vi "OpenScan-20170126-FPGA.vi"() -> ()   [LabVIEW 2015]
uses:
  <vilib>/Platform/TimedLoop/XDataNode/XDataNode.xnode
  <vilib>/Platform/TimedLoop/XDataNode/nitl_modes.ctl
  <vilib>/Platform/TimedLoop/XDataNode/XDNodeRunTimeDep.lvlib
  <vilib>/Platform/TimedLoop/XDataNode/wakeup.ctl
  <vilib>/Platform/TimedLoop/XDataNode/timing_clust.ctl
  <vilib>/rvi/DataTransferAndStorage/Container/XNode/niFpgaContainer.xnode
  <vilib>/eio/EIONode/EIONode.xnode
  <vilib>/rvi/eio/common/nirviEmuTemplateMethod_errors.vi
  <vilib>/rvi/interface/RandomDataEmulation/nirviRandomDataFpgaReadWriteTemplate.vi
  <vilib>/rvi/Memory/Memory_Emulation/niFpgaMemoryEmulationDramWriteAndRequestData.vi
  <vilib>/rvi/Memory/Memory_Emulation/niFpgaMemoryFastEmulationDramWriteAndRequestData.vi
  <vilib>/rvi/Memory/Memory_Emulation/niFpgaMemoryEmulationDramRetrieveData.vi
  <vilib>/rvi/LocalResourceManager/LocalResourceManager.xnode
  <vilib>/rvi/DataTransferAndStorage/Container/Common/niFpgaContainerGetUniqueNameForEmu.vi
  <vilib>/rvi/DataTransferAndStorage/Container/Common/niFpgaContainerSetEmuInfo.vi
  <vilib>/rvi/eio/common/nirviEmuReportErrorAndStop.vi
  <vilib>/rvi/FIFO/Fifo_Resource/nirvififoEmulationRead.vi
  <vilib>/rvi/FIFO/Fifo_Resource/nirvififoEmulationWrite.vi
  <vilib>/rvi/FIFO/Fifo_Resource/nirvififoEmulationClear.vi
panel:
  out "Scan rate(ticks)":u32
  out "loop count":i32
  out "Averaged data address":u32
  out "Averaged image displayed?":bool
  out "Image averaging done?":bool
  in  "Kalman gain":fxp<+,16,1>=0.1015625
  in  "Filter gain":fxp<+,16,0>=0.8000030517578125
  out "Pixel clock":bool
  out "Line clock":bool
  out "Next frame?":bool
  out "Display_frames done":i32
  out "Waveform output frames done":i32
  out "Acquisition frames done":i32
  in  "Frame retrace time":u32 caption="Frame retrace time (ms)"
  out "All waveform output finish?":bool
  in  "Imaging mode":i16(ring)=2 items=["Grab, single frame", "Focus, infinite frames", "Loop, finite frames"]
  in  "Num of frames":i32
  out "Frame Galvo signal write done?":bool
  in  "Total elements":u32
  out "Frame address":u32
  in  "Write Frame Galvo signal?":bool
  in  "max addr":u32=1024
  out "Write DRAM done?":bool
  in  "Write DRAM enable?":bool
  out "Imaging data address":u32
  out "Frame imaging data displayed?":bool
  out "Frame acquisition finish?":bool
  in  "Samples per frame":u32
  in  "Pixel pulse_initial delay":i32
  out "Samples acquired":u32
  in  "Pixel clock_pulse width(tick)":i32
  in  "Resolution":i32
  in  "Num of undershoot":i32
  in  "Elements per line":i32
  out "Request address":u32
  out "Galvo signal readed":u32
  out "Frame waveform output finish?":bool
  out "Data":u32
  in  "Num of elements":u32
  in  "Pixel time (tick)":i32
  # "Waveform generation"
  # "Acquisition"
  # "Kalman filter and image diaplay"
  # "This vi is the FPGA vi for a laser scanning microscope working under photon conuting mode. It \ncontrols scan waveform generation, sychronized data acquisition, Kalman filter of imaging data,\nand transfer processed data to PC for display."
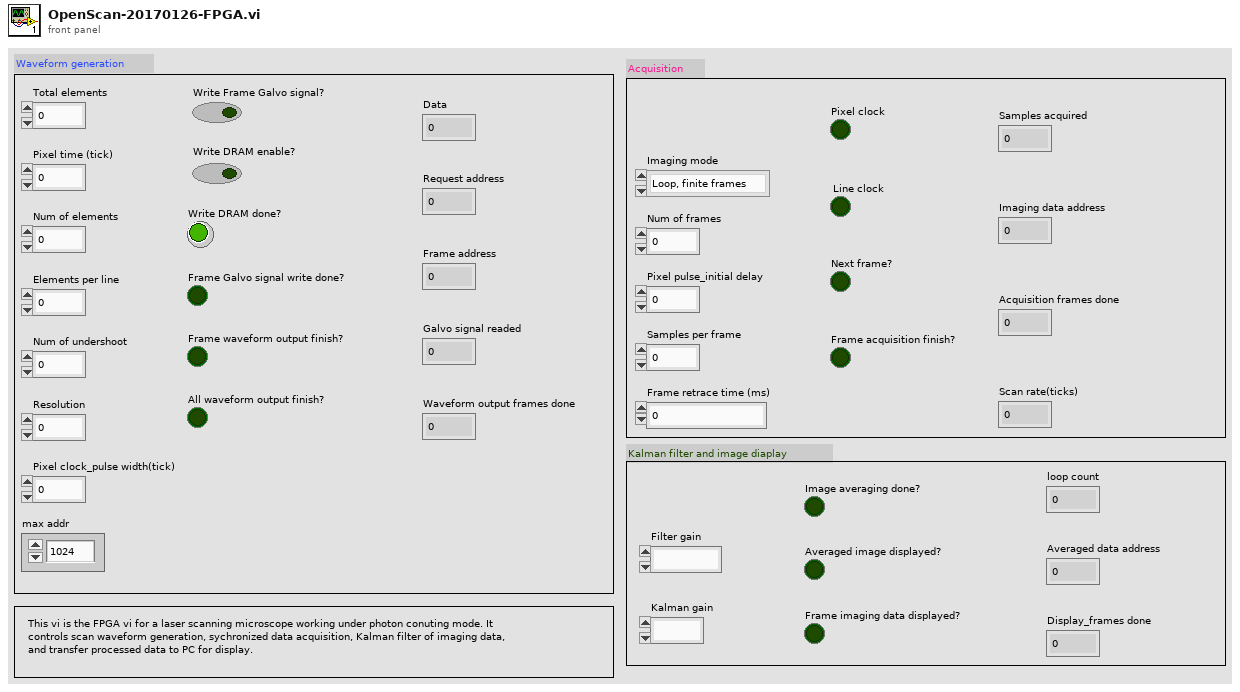
[diagram p1: front panel]
types:
  T1 = typedef "XDNodeRunTimeDep.lvlib/timing_clust.ctl" = cluster{"Expected End [f-1]":u64, "Actual End [f-1]":u64, "Finished Late? [f-1]":bool, "Expected End [i-1]":u64, "Actual End [i-1]":u64, "Finished Late? [i-1]":bool, "Expected Start [i]":u64, "Actual Start [i]":u64, "Expected Start [f]":u64, "Actual Start [f]":u64, "Source Name":string, "Structure Name":string, "Period":i64, "Deadline":i64, "Offset":i64, "Start":i64, "Priority":i32, "Timeout":i32, "Mode":T2, "Wakeup Reason":T3, "Error":errorcluster, "Source Type":string, "Secondary Source Type":string, "Global End Time":u64, "Global Start Time":u64, "Frame Duration":u64, "Iteration Duration":u64, "Assigned CPU":i32, "I/O Scan Engine Mode":u32}
  T2 = typedef "XDNodeRunTimeDep.lvlib/nitl_modes.ctl" = enum32{"No Change", "Process missed periods, maintain original phase", "Discard missed periods, maintain original phase", "Process missed periods, ignore original phase", "Discard missed periods, ignore original phase"}
  T3 = typedef "XDNodeRunTimeDep.lvlib/wakeup.ctl" = enum32{"Normal", "Aborted", "Asynchronous wakeup", "Timing source error", "Timed loop error", "Timeout"}
  T4 = cluster{"Numeric 1":u32, "Numeric 2":u32, "Numeric 3":u32, "Numeric 4":u32, "Numeric 5":u32, "Numeric 6":u32, "Numeric 7":u32, "Numeric 8":u32, "Numeric 9":u32, "Numeric 10":u32, "Numeric 11":u32, "Numeric 12":u32, "Numeric 13":u32, "Numeric 14":u32, "Numeric 15":u32, "Numeric 16":u32}
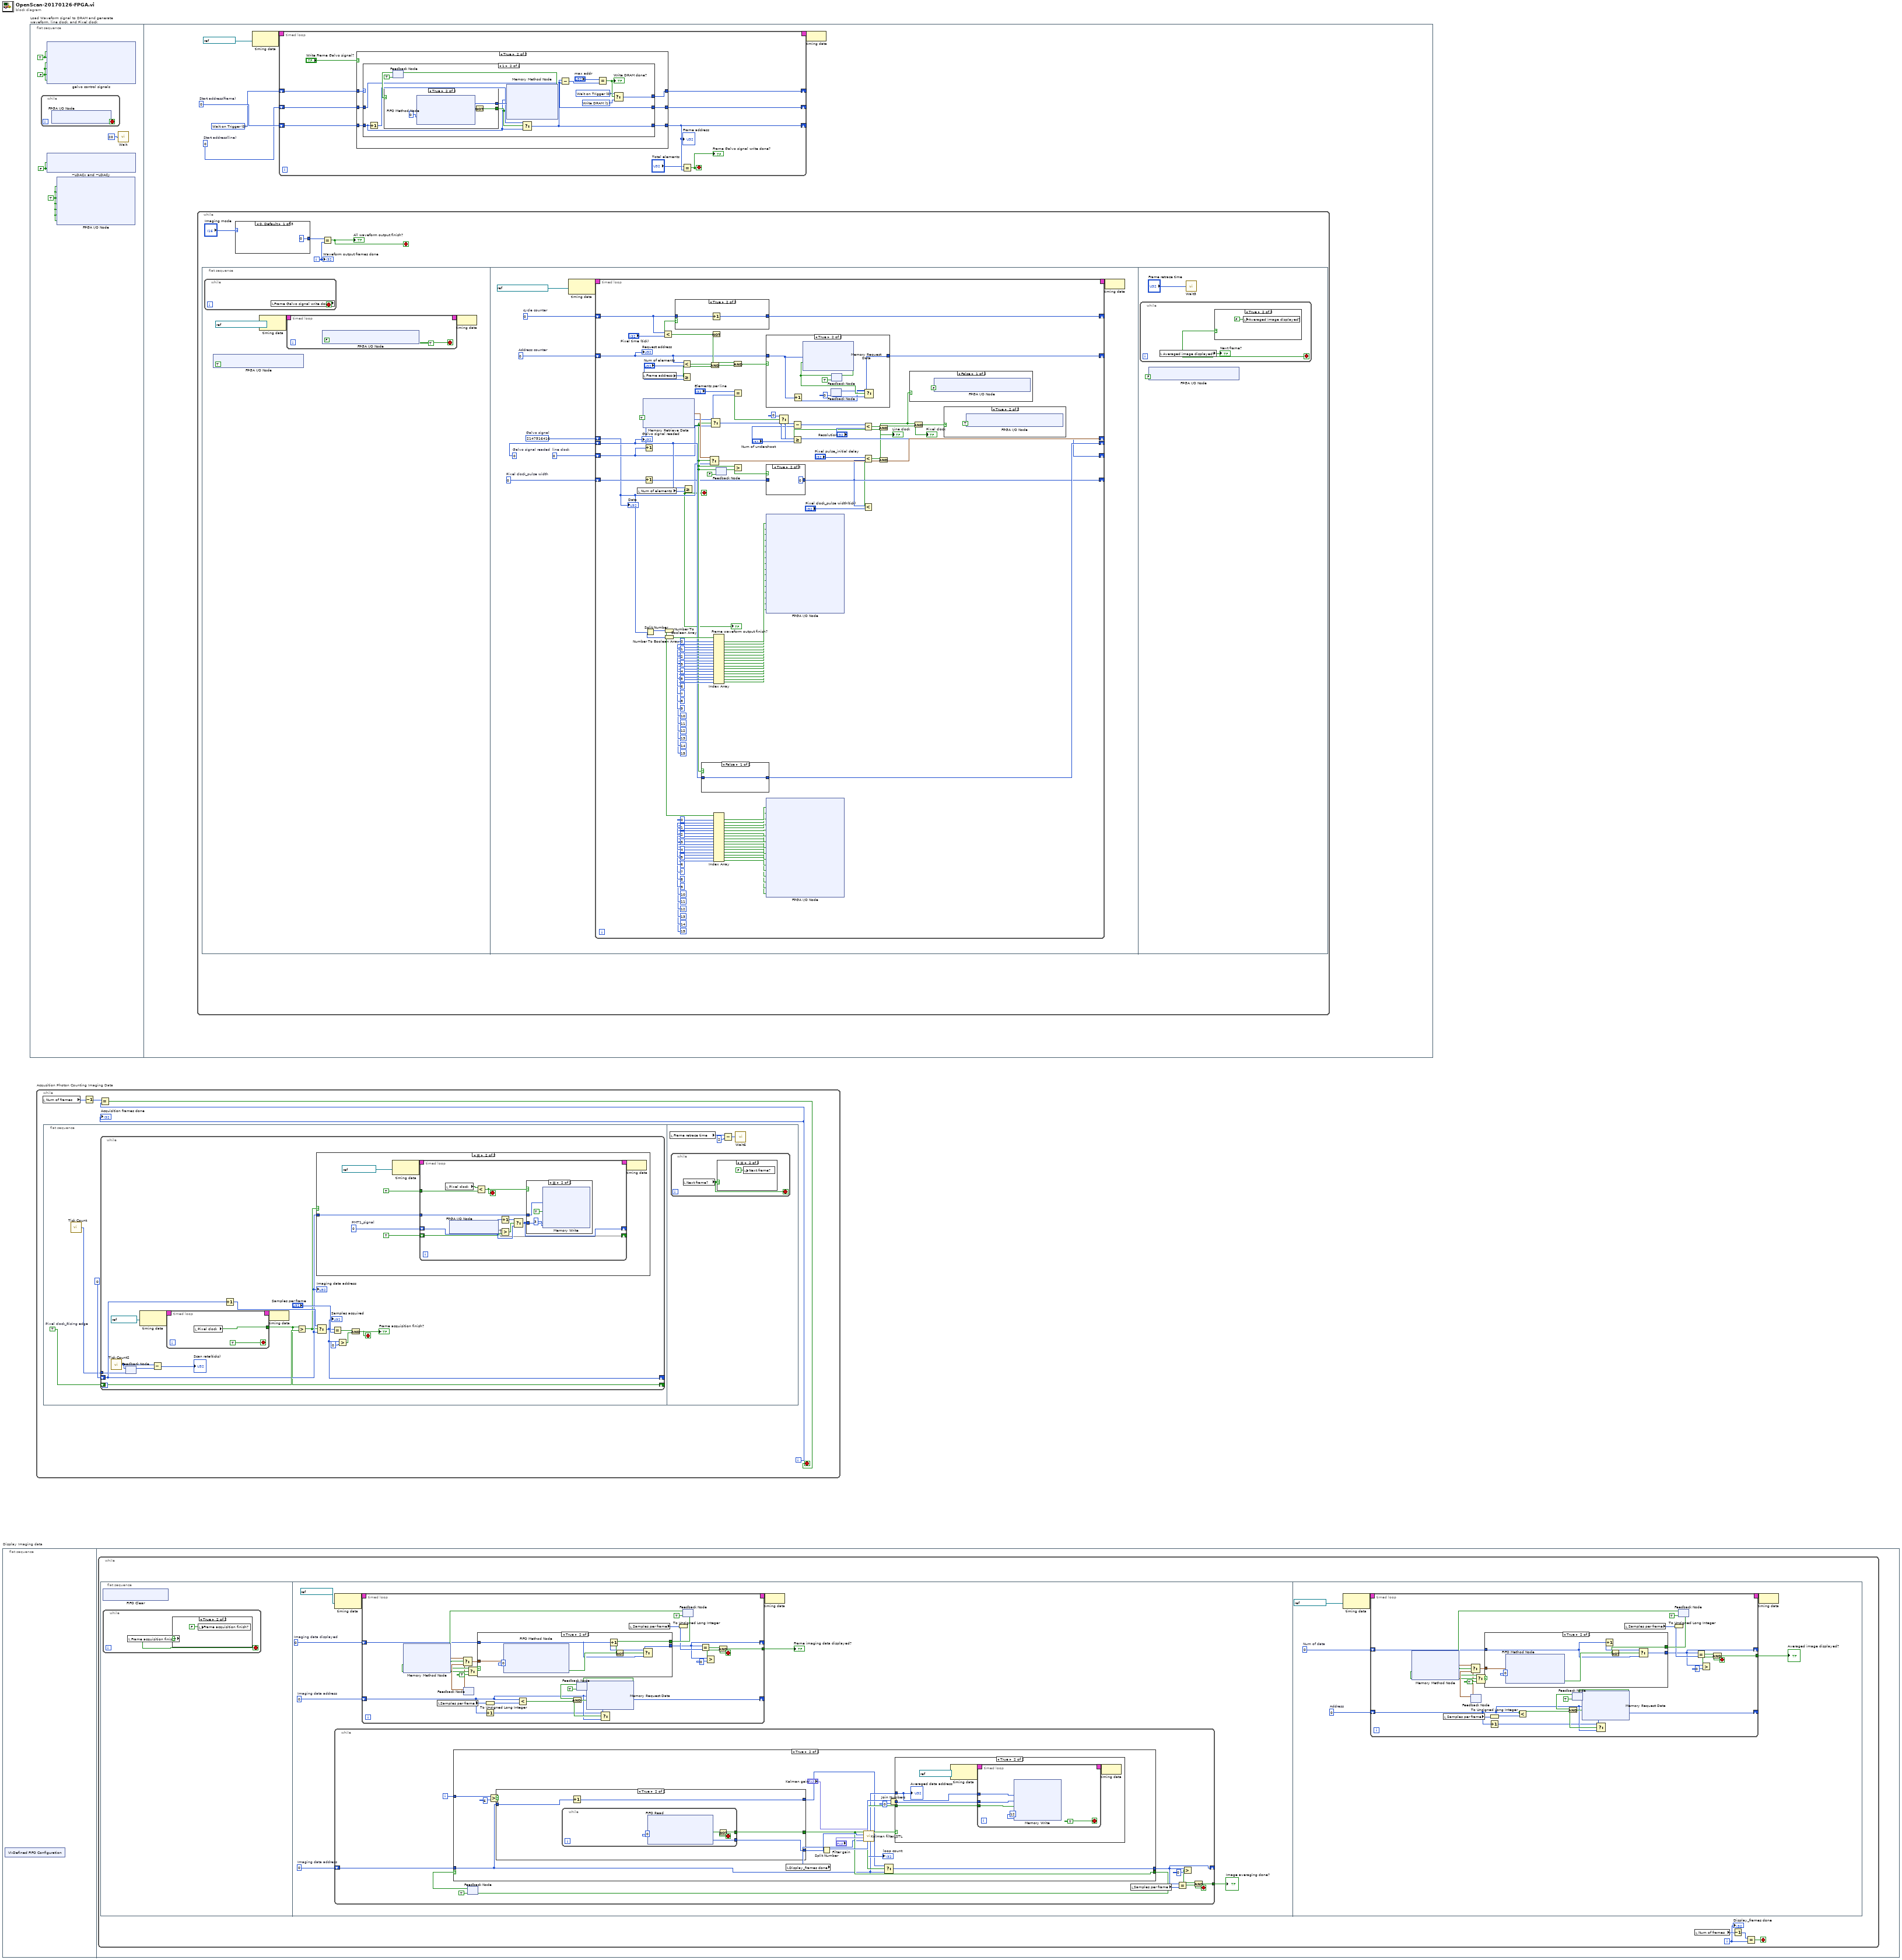
[diagram p0: block diagram]
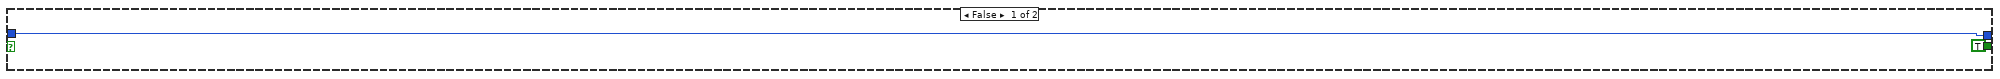
[diagram p6: hidden frame]
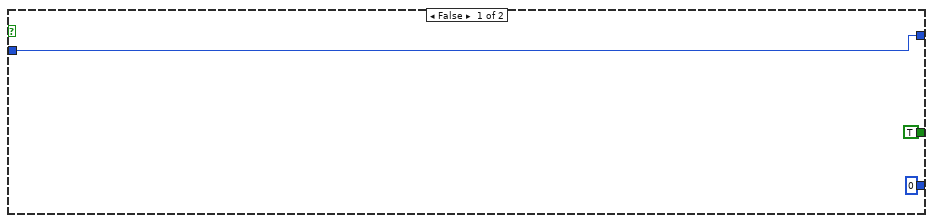
[diagram p7: hidden frame]
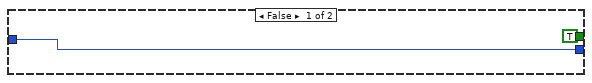
[diagram p9: hidden frame]
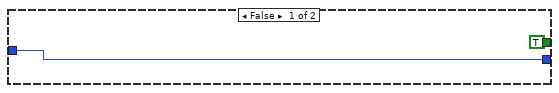
[diagram p10: hidden frame]
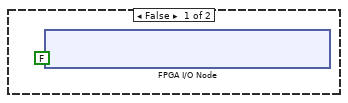
[diagram p11: hidden frame]
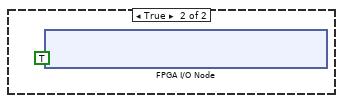
[diagram p13: hidden frame]
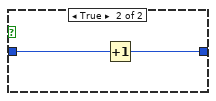
[diagram p14: hidden frame]
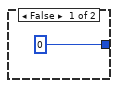
[diagram p16: hidden frame]
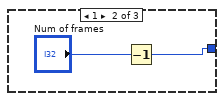
[diagram p18: hidden frame]
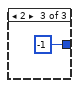
[diagram p19: hidden frame]
diagram:
  n1 = flat-sequence "Display Imaging data" {
    frame #0 {
      n2 = xnode "VI-Defined FIFO Configuration"() -> ()  [unwired: 1 out]
    }
    frame #1 {
      n3 = while {
        i -> [w1]
        stop <- w3 stop-if-true
        n4 = flat-sequence {
          frame #0 {
            n5 = xnode ("FIFO Clear")() -> ()  [unwired: 1 in, 1 out]
            n6 = while {
              stop <- w5 stop-if-true
              n7 = local read "Frame acquisition finish?"() -> (w5:bool)
              n8 = case shown="True" w5 {
                frame False {
                }
                frame True {
                  n9 = local write "Frame acquisition finish?"(FALSE ("Frame acquisition finish?")) -> ()
                }
              }
            }
          }
          frame #1 {
            w8 = u32 0  # Imaging data address
            w11 = u32 0  # Imaging data displayed
            w12 = u32 0  # Imaging data address
            n10 = node-c288(refnum<k21> "DRAM Clock" ("Source Name")) -> (w14:T1)
            n11 = while {
              shift-right: [w21] -> _
              shift-left: w8 -> [w23]
              tunnel: [w18] -> w7
              i -> [w15]
              stop <- w18 stop-if-true
              n12 = feedback #1(TRUE ("Timed Out?")) -> (w24:bool)
              n13 = case shown="True" w24 {
                tunnel: [TRUE ("Timed Out?") w35] -> w25
                tunnel: w23 -> [w26 w29]
                tunnel: [w26 w41] -> w21
                tunnel: w15 -> [_ w32]
                frame False {
                }
                frame True {
                  n14 = Greater?(x=w32, y=6) -> (0:w30:bool)
                  n15 = case shown="True" w30 {
                    tunnel: [u32 0 ("Element") w52] -> w45
                    tunnel: [TRUE w51] -> w35
                    tunnel: w29 -> [w48 w50]
                    tunnel: [w48 w49] -> w28
                    frame False {
                    }
                    frame True {
                      n16 = while {
                        tunnel: [w53] -> w51
                        tunnel: [w54] -> w52
                        stop <- w53 stop-if-true
                        n17 = xnode ("FIFO Read")("超时"=0 ("Timeout")) -> ("元素"=w54:u32, "超时？"=w55:bool)  [unwired: 1 in, 1 out]
                        n18 = Not(x=w55) -> (.not. x?=w53:bool)
                      }
                      n19 = Increment(x=w50) -> (x+1=w49:u32)
                    }
                  }
                  n20 = local read "Display_frames done"() -> (w33:i32)
                  n21 = Split Number(x=w45) -> (hi(x)=w40:u16, lo(x)=w43:u16)
                  n22 = call "Kalman filter_STL.vi"("Previous predicted pixel value"=w40, "Kalman gain"="Kalman gain", "Frame number"=w33, "Filter gain"="Filter gain", "Pixel value"=w43, "Input valid"=w35) -> ("Kalman filter result"=w38:u16, "loop count"=→"loop count":i32, "output valid"=w36:bool)  [unwired: 3 in]
                  n23 = Select(t=w28, s=w36, f=w29) -> (s? t:f=w41:u32)
                  n24 = Join Numbers(hi=w38, lo=u16 0) -> ((hi.lo)=w39:u32)
                  n25 = case shown="True" w36 {
                    tunnel: w36 -> [_ w60]
                    tunnel: w29 -> [_ w59]
                    tunnel: w39 -> [_ w57]
                    frame False {
                    }
                    frame True {
                      n26 = node-c288(refnum<k21> "DRAM Clock" ("Source Name")) -> (w62:T1)
                      n27 = timed-loop {
                        timing: w62 -> [_]
                        timing-out: [_] -> w61
                        tunnel: w57 -> [w67]
                        tunnel: w60 -> [w66]
                        tunnel: w59 -> [w65]
                        stop <- TRUE stop-if-true
                        n28 = xnode ("Memory Write")("地址"=w65, "数据"=w67, "输入有效"=w66, "字节启用"=i64 12 ("Byte Enables")) -> ()  [unwired: 1 in, 2 out]
                      }
                      n29 = node-c288(w61) -> ()
                      "Averaged data address" <- w59
                    }
                  }
                }
              }
              n30 = feedback-in #1(w25) -> ()
              n31 = local read "Samples per frame"() -> (w17:u32)
              n32 = Equal?(x=w21, y=w17) -> (x = y?=w19:bool)
              n33 = Greater?(x=w21, y=u32 0) -> (0:w20:bool)
              n34 = And(x=w20, y=w19) -> (x .and. y?=w18:bool)
            }
            "Image averaging done?" <- w7
            n35 = timed-loop {
              shift-right: [w93] -> _
              shift-left: w12 -> [w95]
              timing: w14 -> [_]
              timing-out: [_] -> w13
              shift-right: [w80] -> _
              shift-left: w11 -> [w83]
              tunnel: [w75] -> w9
              stop <- w75 stop-if-true
              n36 = local read "Samples per frame"() -> (w100:u32)
              n37 = feedback #2() -> (w87:T4)  [unwired: 1 in]
              n38 = To Unsigned Long Integer(number=w100) -> (unsigned 32bit integer=w82:u32)
              n39 = Increment(x=w95) -> (x+1=w94:u32)
              n40 = Less?(x=w95, y=w82) -> (x < y?=w99:bool)
              n41 = feedback #3(TRUE ("Ready for Input")) -> (w97:bool)
              n42 = And(x=w97, y=w99) -> (x .and. y?=w96:bool)
              n43 = xnode ("Memory Request Data")("地址"=w95, "输入有效"=w96) -> ("输入就绪"=w98:bool)  [unwired: 1 in, 1 out]
              n44 = feedback-in #3(w98) -> ()
              n45 = Select(t=w94, s=w96, f=w95) -> (s? t:f=w93:u32)
              n46 = local read "Samples per frame"() -> (w92:u32)
              n47 = To Unsigned Long Integer(number=w92) -> (unsigned 32bit integer=w81:u32)
              n48 = feedback #4(TRUE) -> (w86:bool)
              n49 = xnode ("Memory Method Node")("输出就绪"=w86) -> ("数据"=w91:T4, "输出有效"=w84:bool)  [unwired: 1 in, 1 out]
              n50 = Select(t=w91, s=w86, f=w87) -> (s? t:f=w74:T4)
              n51 = feedback-in #2(w74) -> ()
              n52 = Select(t=w84, s=w86, f=TRUE) -> (s? t:f=w90:bool)
              n53 = case shown="True" w90 {
                tunnel: [TRUE w106] -> w89
                tunnel: w74 -> [_ w103]
                tunnel: w83 -> [w101 w105]
                tunnel: [w101 w104] -> w80
                frame False {
                }
                frame True {
                  n54 = xnode ("FIFO Method Node")("元素"=w103, "超时"=0 ("Timeout")) -> ("超时？"=w108:bool)  [unwired: 1 in, 1 out]
                  n55 = Increment(x=w105) -> (x+1=w107:u32)
                  n56 = Not(x=w108) -> (.not. x?=w106:bool)
                  n57 = Select(t=w107, s=w106, f=w105) -> (s? t:f=w104:u32)
                }
              }
              n58 = feedback-in #4(w89) -> ()
              n59 = Equal?(x=w80, y=w81) -> (x = y?=w77:bool)
              n60 = Greater?(x=w80, y=u32 0) -> (0:w78:bool)
              n61 = And(x=w77, y=w78) -> (x .and. y?=w75:bool)
            }
            "Frame imaging data displayed?" <- w9
            n62 = node-c288(w13) -> ()
          }
          frame #2 {
            w118 = u32 0  # Address
            w119 = u32 0  # Num of data
            n63 = node-c288(refnum<k21> "DRAM Clock" ("Source Name")) -> (w121:T1)
            n64 = timed-loop {
              shift-right: [w141] -> _
              shift-left: w118 -> [w143]
              timing: w121 -> [_]
              timing-out: [_] -> w120
              shift-right: [w128] -> _
              shift-left: w119 -> [w131]
              tunnel: [w123] -> w117
              stop <- w123 stop-if-true
              n65 = local read "Samples per frame"() -> (w148:u32)
              n66 = feedback #5() -> (w135:T4)  [unwired: 1 in]
              n67 = To Unsigned Long Integer(number=w148) -> (unsigned 32bit integer=w130:u32)
              n68 = Increment(x=w143) -> (x+1=w142:u32)
              n69 = Less?(x=w143, y=w130) -> (x < y?=w147:bool)
              n70 = feedback #6(TRUE ("Ready for Input")) -> (w145:bool)
              n71 = And(x=w145, y=w147) -> (x .and. y?=w144:bool)
              n72 = xnode ("Memory Request Data")("地址"=w143, "输入有效"=w144) -> ("输入就绪"=w146:bool)  [unwired: 1 in, 1 out]
              n73 = feedback-in #6(w146) -> ()
              n74 = Select(t=w142, s=w144, f=w143) -> (s? t:f=w141:u32)
              n75 = local read "Samples per frame"() -> (w140:u32)
              n76 = To Unsigned Long Integer(number=w140) -> (unsigned 32bit integer=w129:u32)
              n77 = feedback #7(TRUE) -> (w134:bool)
              n78 = xnode ("Memory Method Node")("输出就绪"=w134) -> ("数据"=w139:T4, "输出有效"=w132:bool)  [unwired: 1 in, 1 out]
              n79 = Select(t=w139, s=w134, f=w135) -> (s? t:f=w122:T4)
              n80 = feedback-in #5(w122) -> ()
              n81 = Select(t=w132, s=w134, f=TRUE) -> (s? t:f=w138:bool)
              n82 = case shown="True" w138 {
                tunnel: [TRUE w154] -> w137
                tunnel: w122 -> [_ w151]
                tunnel: w131 -> [w149 w153]
                tunnel: [w149 w152] -> w128
                frame False {
                }
                frame True {
                  n83 = xnode ("FIFO Method Node")("元素"=w151, "超时"=0 ("Timeout")) -> ("超时？"=w156:bool)  [unwired: 1 in, 1 out]
                  n84 = Increment(x=w153) -> (x+1=w155:u32)
                  n85 = Not(x=w156) -> (.not. x?=w154:bool)
                  n86 = Select(t=w155, s=w154, f=w153) -> (s? t:f=w152:u32)
                }
              }
              n87 = feedback-in #7(w137) -> ()
              n88 = Equal?(x=w128, y=w129) -> (x = y?=w125:bool)
              n89 = Greater?(x=w128, y=u32 0) -> (0:w126:bool)
              n90 = And(x=w125, y=w126) -> (x .and. y?=w123:bool)
            }
            "Averaged image displayed?" <- w117
            n91 = node-c288(w120) -> ()
          }
        }
        n92 = local read "Num of frames"() -> (w4:i32)
        n93 = Decrement(x=w4) -> (x-1=w2:i32)
        n94 = Equal?(x=w2, y=w1) -> (x = y?=w3:bool)
        "Display_frames done" <- w1
      }
    }
  }
  n95 = flat-sequence "Load Waveform signal to DRAM and generate waveform, line clock, and Pixel clock" {
    frame #0 {
      w166 = FALSE ("_LDACx")
      w168 = FALSE ("_CSx")
      w167 = TRUE ("_CLRx")
      w164 = TRUE ("IO Module\\DDCA_DIO8-15_WE")
      n96 = while {
        stop <- w169 stop-if-true
        n97 = xnode "FPGA I/O Node"() -> ("IO Module IO Enabled"=w169)  [unwired: 1 in, 1 out]
      }
      n98 = xnode "galvo control signals"("IO Module\\CLRx(DDCB_DIO0_WRITE)"=w167, "IO Module\\CLRy(DDCB_DIO1_WRITE)"=w167, "IO Module\\CSx(DDCB_DIO2_WRITE)"=w168, "IO Module\\CSy(DDCB_DIO3_WRITE)"=w168, "IO Module\\R_Wx(DDCB_DIO4_WRITE)"=w168, "IO Module\\R_Wy(DDCB_DIO5_WRITE)"=w168) -> ()  [unwired: 6 in, 6 out]
      n99 = xnode "~LDACx and ~LDACy"("IO Module\\LDAx(DDCB_DIO6_WRITE)"=w166, "IO Module\\LDAy(DDCB_DIO7_WRITE)"=w166) -> ()  [unwired: 2 in, 2 out]
      n100 = xnode "FPGA I/O Node"("IO Module\\DDCA_DIO8-15_WE"=w164, "IO Module\\DDCA_DIO16-23_WE"=w164, "IO Module\\DDCB_DIO8-15_WE"=w164, "IO Module\\DDCB_DIO16-23_WE"=w164, "IO Module\\DDCB_DIO0-7_WE"=w164, "IO Module\\DDCB_PFI_WE"=w164, "IO Module\\DDCA_PFI_WE"=w164) -> ()  [unwired: 7 in, 7 out]
      n101 = call "Wait"("Count(mSec)"=u32 20) -> ()  [unwired: 1 out]
    }
    frame #1 {
      w170 = 0 items=["Wait on Trigger", "Write DRAM"]
      w172 = u32 0  # Start address(line)
      w173 = u32 0  # Start address(frame)
      n102 = while {
        i -> [w177]
        stop <- w176 stop-if-true
        n103 = flat-sequence {
          frame #0 {
            n104 = while {
              stop <- w192 stop-if-true
              n105 = local read "Frame Galvo signal write done?"() -> (w192:bool)
            }
            n106 = xnode "FPGA I/O Node"("IO Module\\Shutter(DDCA_PFI1_WRITE)"=TRUE ("IO Module\\Shutter(DDCA_PFI1_WRITE)")) -> ()  [unwired: 1 in, 1 out]
            n107 = node-c288(refnum<k21> "40 MHz Onboard Clock" ("Source Name")) -> (w182:T1)
            n108 = timed-loop {
              timing: w182 -> [_]
              timing-out: [_] -> w181
              stop <- TRUE stop-if-true
              n109 = xnode "FPGA I/O Node"("IO Module\\(Pixel clock)DDCB_PFI3_WRITE"=FALSE ("IO Module\\(Pixel clock)DDCB_PFI3_WRITE")) -> ()  [unwired: 1 in, 1 out]
            }
            n110 = node-c288(w181) -> ()
          }
          frame #1 {
            w193 = 0  # Pixel clock_pulse width
            w194 = 0  # line clock
            w195 = u32 0  # Galvo signal readed
            w197 = u32 2147516416  # Galvo signal
            w198 = u32 0  # Address counter
            w196 = 0  # cycle counter
            n111 = node-c288(refnum<k21> "40 MHz Onboard Clock" ("Source Name")) -> (w201:T1)
            n112 = timed-loop {
              timing: w201 -> [_]
              timing-out: [_] -> w200
              shift-right: [w245] -> _
              shift-left: w198 -> [w231]
              shift-right: [w244] -> _
              shift-left: w197 -> [w208]
              shift-right: [w237] -> _
              shift-left: w196 -> [w235]
              shift-right: [w243] -> _
              shift-left: w195 -> [w232]
              shift-right: [w224] -> _
              shift-left: w194 -> [w229]
              shift-right: [w212] -> _
              shift-left: w193 -> [w218]
              stop <- w202 stop-if-true
              n113 = local read "Num of elements"() -> (w241:u32)
              n114 = local read "Frame address"() -> (w203:u32)
              n115 = xnode ("Memory Retrieve Data")("输出就绪"=TRUE ("Ready for Output")) -> ("数据"=w250:T4, "输出有效"=w217:bool)  [unwired: 1 in, 1 out]
              n116 = Increment(x=w229) -> (x+1=w230:i32)
              n117 = Increment(x=w218) -> (x+1=w213:i32)
              n118 = Split Number(x=w208) -> (hi(x)=w248:u16, lo(x)=w249:u16)
              n119 = Less?(x=w235, y="Pixel time (tick)") -> (x < y?=w234:bool)
              n120 = Number To Boolean Array(number=w248) -> (Boolean array=w316:bool[])
              n121 = Number To Boolean Array(number=w249) -> (Boolean array=w251:bool[])
              n122 = case shown="True" w234 {
                tunnel: w235 -> [_ w337]
                tunnel: [0 w336] -> w237
                frame False {
                }
                frame True {
                  n123 = Increment(x=w337) -> (x+1=w336:i32)
                }
              }
              n124 = Less?(x=w231, y="Num of elements") -> (x < y?=w247:bool)
              n125 = Greater Or Equal?(x=w203, y="Num of elements") -> (x >= y?=w246:bool)
              n126 = Greater Or Equal?(x=w232, y=w241) -> (x >= y?=w202:bool)
              "Frame waveform output finish?" <- w202
              n127 = case shown="False" w217 {
                tunnel: w232 -> [w323 w325]
                tunnel: [w323 w324] -> w243
                frame False {
                }
                frame True {
                  n128 = Increment(x=w325) -> (x+1=w324:u32)
                }
              }
              n129 = Select(t=w250, s=w217, f=w208) -> (s? t:f=w244:T4)
              n130 = And(x=w247, y=w246) -> (x .and. y?=w239:bool)
              n131 = Select(t=w230, s=w217, f=w229) -> (s? t:f=w226:i32)
              n132 = Not(x=w234) -> (.not. x?=w233:bool)
              n133 = Index Array(array=w251, index #1=0 ("index"), index #2=1 ("index"), index #3=2 ("index"), index #4=3 ("index"), index #5=4 ("index"), index #6=5 ("index"), index #7=6 ("index"), index #8=7 ("index"), index #9=8 ("index"), index #10=9 ("index"), index #11=10 ("index"), index #12=11 ("index"), index #13=12 ("index"), index #14=13 ("index"), index #15=14 ("index"), index #16=15 ("index")) -> (element #1=w267:bool, element #2=w266:bool, element #3=w265:bool, element #4=w264:bool, element #5=w263:bool, element #6=w262:bool, element #7=w261:bool, element #8=w260:bool, element #9=w259:bool, element #10=w258:bool, element #11=w257:bool, element #12=w256:bool, element #13=w255:bool, element #14=w254:bool, element #15=w253:bool, element #16=w252:bool)
              n134 = Index Array(array=w316, index #1=0 ("index"), index #2=1 ("index"), index #3=2 ("index"), index #4=3 ("index"), index #5=4 ("index"), index #6=5 ("index"), index #7=6 ("index"), index #8=7 ("index"), index #9=8 ("index"), index #10=9 ("index"), index #11=10 ("index"), index #12=11 ("index"), index #13=12 ("index"), index #14=13 ("index"), index #15=14 ("index"), index #16=15 ("index")) -> (element #1=w299:bool, element #2=w298:bool, element #3=w297:bool, element #4=w296:bool, element #5=w295:bool, element #6=w294:bool, element #7=w293:bool, element #8=w292:bool, element #9=w291:bool, element #10=w290:bool, element #11=w289:bool, element #12=w288:bool, element #13=w287:bool, element #14=w286:bool, element #15=w285:bool, element #16=w284:bool)
              n135 = feedback-in #8(w217) -> ()
              n136 = feedback #8(FALSE ("Output Valid")) -> (w216:bool)
              n137 = And(x=w233, y=w239) -> (x .and. y?=w238:bool)
              n138 = Equal?(x="Elements per line", y=w226) -> (x = y?=w227:bool)
              n139 = Greater?(x=w217, y=w216) -> (0:w207:bool)
              n140 = case shown="True" w238 {
                tunnel: w231 -> [w326 w333]
                tunnel: [w326 w330] -> w245
                frame False {
                }
                frame True {
                  n141 = Increment(x=w333) -> (x+1=w329:u32)
                  n142 = feedback #9(u32 0) -> (w331:u32)
                  n143 = feedback #10(TRUE ("Ready for Input")) -> (w332:bool)
                  n144 = xnode ("Memory Request Data")("地址"=w333, "输入有效"=w332) -> ("输入就绪"=w334:bool)  [unwired: 1 in, 1 out]
                  n145 = feedback-in #10(w334) -> ()
                  n146 = Select(t=w329, s=w332, f=w331) -> (s? t:f=w330:u32)
                  n147 = feedback-in #9(w330) -> ()
                }
              }
              n148 = case shown="True" w207 {
                tunnel: w213 -> [w319 _]
                tunnel: [w319 0] -> w212
                frame False {
                }
                frame True {
                }
              }
              n149 = xnode "FPGA I/O Node"("IO Module\\DDCB_DIO8_WRITE"=w267, "IO Module\\DDCB_DIO9_WRITE"=w266, "IO Module\\DDCB_DIO10_WRITE"=w265, "IO Module\\DDCB_DIO11_WRITE"=w264, "IO Module\\DDCB_DIO12_WRITE"=w263, "IO Module\\DDCB_DIO13_WRITE"=w262, "IO Module\\DDCB_DIO14_WRITE"=w261, "IO Module\\DDCB_DIO15_WRITE"=w260, "IO Module\\DDCB_DIO16_WRITE"=w259, "IO Module\\DDCB_DIO17_WRITE"=w258, "IO Module\\DDCB_DIO18_WRITE"=w257, "IO Module\\DDCB_DIO19_WRITE"=w256, "IO Module\\DDCB_DIO20_WRITE"=w255, "IO Module\\DDCB_DIO21_WRITE"=w254, "IO Module\\DDCB_DIO22_WRITE"=w253, "IO Module\\DDCB_DIO23_WRITE"=w252) -> ()  [unwired: 16 in, 16 out]
              n150 = xnode "FPGA I/O Node"("IO Module\\DDCA_DIO8_WRITE"=w299, "IO Module\\DDCA_DIO9_WRITE"=w298, "IO Module\\DDCA_DIO10_WRITE"=w297, "IO Module\\DDCA_DIO11_WRITE"=w296, "IO Module\\DDCA_DIO12_WRITE"=w295, "IO Module\\DDCA_DIO13_WRITE"=w294, "IO Module\\DDCA_DIO14_WRITE"=w293, "IO Module\\DDCA_DIO15_WRITE"=w292, "IO Module\\DDCA_DIO16_WRITE"=w291, "IO Module\\DDCA_DIO17_WRITE"=w290, "IO Module\\DDCA_DIO18_WRITE"=w289, "IO Module\\DDCA_DIO19_WRITE"=w288, "IO Module\\DDCA_DIO20_WRITE"=w287, "IO Module\\DDCA_DIO21_WRITE"=w286, "IO Module\\DDCA_DIO22_WRITE"=w285, "IO Module\\DDCA_DIO23_WRITE"=w284) -> ()  [unwired: 16 in, 16 out]
              n151 = Select(t=0, s=w227, f=w226) -> (s? t:f=w224:i32)
              n152 = Subtract(x=w224, y="Num of undershoot") -> (x-y=w222:i32)
              n153 = Greater Or Equal?(x=w224, y="Num of undershoot") -> (x >= y?=w219:bool)
              n154 = Less?(x=w222, y="Resolution") -> (x < y?=w220:bool)
              n155 = Less?(x="Pixel pulse_initial delay", y=w212) -> (x < y?=w210:bool)
              n156 = Less?(x=w212, y="Pixel clock_pulse width(tick)") -> (x < y?=w209:bool)
              n157 = And(x=w210, y=w209) -> (x .and. y?=w205:bool)
              n158 = And(x=w220, y=w219) -> (x .and. y?=w206:bool)
              "Line clock" <- w206
              n159 = case shown="False" w206 {
                frame False {
                  n160 = xnode "FPGA I/O Node"("IO Module\\Line clock(DDCB_PFI2_WRITE)"=FALSE ("IO Module\\Line clock(DDCB_PFI2_WRITE)")) -> ()  [unwired: 1 in, 1 out]
                }
                frame True {
                  n161 = xnode "FPGA I/O Node"("IO Module\\Line clock(DDCB_PFI2_WRITE)"=TRUE ("IO Module\\Line clock(DDCB_PFI2_WRITE)")) -> ()  [unwired: 1 in, 1 out]
                }
              }
              n162 = And(x=w206, y=w205) -> (x .and. y?=w204:bool)
              "Pixel clock" <- w204
              n163 = case shown="True" w204 {
                frame False {
                  n164 = xnode "FPGA I/O Node"("IO Module\\(Pixel clock)DDCB_PFI3_WRITE"=FALSE ("IO Module\\(Pixel clock)DDCB_PFI3_WRITE")) -> ()  [unwired: 1 in, 1 out]
                }
                frame True {
                  n165 = xnode "FPGA I/O Node"("IO Module\\(Pixel clock)DDCB_PFI3_WRITE"=TRUE ("IO Module\\(Pixel clock)DDCB_PFI3_WRITE")) -> ()  [unwired: 1 in, 1 out]
                }
              }
              "Galvo signal readed" <- w232
              "Request address" <- w231
              "Data" <- w208
            }
            n166 = node-c288(w200) -> ()
          }
          frame #2 {
            n167 = while {
              stop <- w346 stop-if-true
              n168 = local read "Averaged image displayed?"() -> (w346:bool)
              "Next frame?" <- w346
              n169 = case shown="True" w346 {
                frame False {
                }
                frame True {
                  n170 = local write "Averaged image displayed?"(FALSE ("Frame imaging data displayed?")) -> ()
                }
              }
            }
            n171 = xnode "FPGA I/O Node"("IO Module\\Shutter(DDCA_PFI1_WRITE)"=FALSE ("IO Module\\Shutter(DDCA_PFI1_WRITE)")) -> ()  [unwired: 1 in, 1 out]
            n172 = call "Wait3"("Count(mSec)"="Frame retrace time") -> ()  [unwired: 1 out]
          }
        }
        n173 = case shown="0, Default" "Imaging mode" {
          tunnel: [0 w349 -1 ("Num of frames")] -> w178
          frame 0, Default {
          }
          frame 1 {
            n174 = Decrement(x="Num of frames") -> (x-1=w349:i32)
          }
          frame 2 {
          }
        }
        n175 = Equal?(x=w178, y=w177) -> (x = y?=w176:bool)
        "All waveform output finish?" <- w176
        "Waveform output frames done" <- w177
      }
      n176 = node-c288(refnum<k21> "DRAM Clock" ("Source Name")) -> (w175:T1)
      n177 = timed-loop {
        timing: w175 -> [_]
        timing-out: [_] -> w174
        shift-right: [w356] -> _
        shift-left: w170 -> [w358]
        shift-right: [w355] -> _
        shift-left: w172 -> [w359]
        shift-right: [w354] -> _
        shift-left: w173 -> [w357]
        stop <- w352 stop-if-true
        n178 = case shown="True" "Write Frame Galvo signal?" {
          tunnel: w358 -> [w363 w369]
          tunnel: w357 -> [w362 w368]
          tunnel: w359 -> [w361 w367]
          tunnel: [w363 w366] -> w356
          tunnel: [w362 w365] -> w354
          tunnel: [w361 w364] -> w355
          frame False {
          }
          frame True {
            n179 = case shown="1" w369 {
              tunnel: w368 -> [w374 w384]
              tunnel: [w374 w382] -> w365
              tunnel: [w376 w388] -> w366
              tunnel: w367 -> [w373 w383]
              tunnel: [w372 w383] -> w364
              frame 0, Default {
                w370 = 0 items=["Wait on Trigger", "Write DRAM"]
                w371 = 1 items=["Wait on Trigger", "Write DRAM"]
                n180 = Select(t=w371, s="Write DRAM enable?", f=w370) -> (s? t:f=w376:i32)
                n181 = case shown="False" "Write DRAM enable?" {
                  tunnel: w374 -> [_ w378]
                  tunnel: w373 -> [w377 _]
                  tunnel: [w377 w378] -> w372
                  frame False {
                  }
                  frame True {
                  }
                }
              }
              frame 1 {
                w379 = 1 items=["Wait on Trigger", "Write DRAM"]
                w380 = 0 items=["Wait on Trigger", "Write DRAM"]
                n182 = Increment(x=w384) -> (x+1=w390:u32)
                n183 = feedback #11(TRUE ("Ready for Input")) -> (w391:bool)
                n184 = case shown="True" w391 {
                  tunnel: [FALSE w397] -> w385
                  tunnel: [u32 0 ("Element") w396] -> w393
                  frame False {
                  }
                  frame True {
                    n185 = xnode ("FIFO Method Node")("超时"=0 ("Timeout")) -> ("元素"=w396:u32, "超时？"=w398:bool)  [unwired: 1 in, 1 out]
                    n186 = Not(x=w398) -> (.not. x?=w397:bool)
                  }
                }
                n187 = xnode ("Memory Method Node")("地址"=w384, "数据"=w393, "输入有效"=w385) -> ("输入就绪"=w392:bool)  [unwired: 1 in, 1 out]
                n188 = feedback-in #11(w392) -> ()
                n189 = Select(t=w390, s=w385, f=w384) -> (s? t:f=w382:u32)
                n190 = Subtract(x=w382, y=w383) -> (x-y=w386:u32)
                n191 = Equal?(x="max addr", y=w386) -> (x = y?=w387:bool)
                "Write DRAM done?" <- w387
                n192 = Select(t=w380, s=w387, f=w379) -> (s? t:f=w388:i32)
              }
            }
          }
        }
        "Frame address" <- w354
        n193 = Equal?(x="Total elements", y=w354) -> (x = y?=w352:bool)
        "Frame Galvo signal write done?" <- w352
      }
      n194 = node-c288(w174) -> ()
    }
  }
  n195 = while "Acqusition Photon Counting Imaging Data" {
    i -> [w407]
    stop <- w408 stop-if-true
    n196 = local read "Num of frames"() -> (w409:i32)
    n197 = flat-sequence {
      frame #0 {
        w412 = TRUE  # Pixel clock_Rising edge
        n198 = call "Tick Count"() -> ("Tick Count(Ticks)"=w410:u32)
        n199 = while {
          shift-right: [w417] -> _
          shift-left: w412 -> [w425]
          shift-right: [w423] -> _
          shift-left: u32 0 -> [w424]
          tunnel: w410 -> [w413]
          stop <- w421 stop-if-true
          n200 = call "Tick Count2"() -> ("Tick Count(Ticks)"=w415:u32)
          n201 = feedback-in #12(w415) -> ()
          n202 = feedback #12(w413) -> (w414:u32)
          n203 = node-c288(refnum<k21> "280MHz" ("Source Name")) -> (w420:T1)
          n204 = Subtract(x=w415, y=w414) -> (x-y=→"Scan rate(ticks)":u32)
          n205 = timed-loop {
            timing: w420 -> [_]
            timing-out: [_] -> w419
            tunnel: [w431] -> w417
            stop <- TRUE stop-if-true
            n206 = local read "Pixel clock"() -> (w431:bool)
          }
          n207 = Increment(x=w424) -> (x+1=w426:u32)
          n208 = node-c288(w419) -> ()
          n209 = Greater?(x=w417, y=w425) -> (0:w422:bool)
          n210 = Select(t=w426, s=w422, f=w424) -> (s? t:f=w423:u32)
          "Samples acquired" <- w423
          n211 = case shown="真" w422 {
            tunnel: w424 -> [_ w440]
            frame False {
            }
            frame True {
              w443 = u16 0  # PMT1_signal
              n212 = node-c288(refnum<k21> "DRAM Clock" ("Source Name")) -> (w445:T1)
              n213 = timed-loop {
                timing: w445 -> [_]
                timing-out: [_] -> w444
                shift-right: [w446] -> _
                shift-left: w443 -> [w455]
                shift-right: [w452] -> _
                shift-left: TRUE ("y") -> [w453]
                tunnel: TRUE -> [w450]
                tunnel: w440 -> [w447]
                stop <- w448 stop-if-true
                n214 = local read "Pixel clock"() -> (w449:bool)
                n215 = xnode "FPGA I/O Node"() -> ("IO Module\\PMT1"=w452)  [unwired: 1 in, 1 out]
                n216 = Less?(x=w449, y=w450) -> (x < y?=w448:bool)
                n217 = Increment(x=w455) -> (x+1=w454:u16)
                n218 = Greater?(x=w452, y=w453) -> (0:w451:bool)
                n219 = Select(t=w454, s=w451, f=w455) -> (s? t:f=w446:u16)
                n220 = case shown="真" w448 {
                  tunnel: w447 -> [_ w459]
                  tunnel: w446 -> [_ w458]
                  frame False {
                  }
                  frame True {
                    n221 = xnode ("Memory Write")("地址"=w459, "数据"=w458, "输入有效"=TRUE ("Input Valid"), "字节启用"=i64 3 ("Byte Enables")) -> ()  [unwired: 1 in, 2 out]
                  }
                }
              }
              n222 = node-c288(w444) -> ()
            }
          }
          n223 = Equal?(x=w423, y="Samples per frame") -> (x = y?=w427:bool)
          n224 = Greater?(x=w423, y=u32 0) -> (0:w428:bool)
          n225 = And(x=w427, y=w428) -> (x .and. y?=w421:bool)
          "Frame acquisition finish?" <- w421
          "Imaging data address" <- w424
        }
      }
      frame #1 {
        n226 = local read "Frame retrace time"() -> (w468:u32)
        n227 = while {
          stop <- w469 stop-if-true
          n228 = local read "Next frame?"() -> (w469:bool)
          n229 = case shown="真" w469 {
            frame False {
            }
            frame True {
              n230 = local write "Next frame?"(FALSE ("Next frame?")) -> ()
            }
          }
        }
        n231 = Subtract(x=w468, y=u32 2) -> (x-y=w466:u32)
        n232 = call "Wait6"("Count(mSec)"=w466) -> ()  [unwired: 1 out]
      }
    }
    n233 = Decrement(x=w409) -> (x-1=w406:i32)
    n234 = Equal?(x=w406, y=w407) -> (x = y?=w408:bool)
    "Acquisition frames done" <- w407
  }
